vi "GetPlane.vi"(0 "Image In":T1 {"Dialogs" format="%.0b"}) -> (1 "Blue Plane Out":T1 {"Dialogs" format="%.0b"}, 2 "Green Plane Out":T1 {"Dialogs" format="%.0b"}, 3 "Red Plane Out":T1 {"Dialogs" format="%.0b"})   [LabVIEW 2024]
doc: "This VI takes as a 24 bit images as an input and will output three 8 bit channels, one each for Red, Green, and Blue."
uses:
  <userlib>/ImageProcessing/QTLIB_2595_LV86/QT_Image.ctl
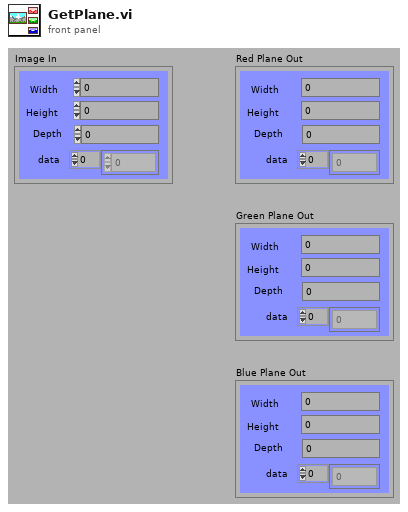
[diagram p1: front panel]
types:
  T1 = typedef "QT_Image.ctl" = cluster{"Width":i32, "Height":i32, "Depth":i32, "data":u8[], "Compressed data":u8[], "Color table":u32[], "Duration":i32, "Options":i32, "Timestamp":i32, "ID":i32, "Reserved":i32, "Dialogs":u32}
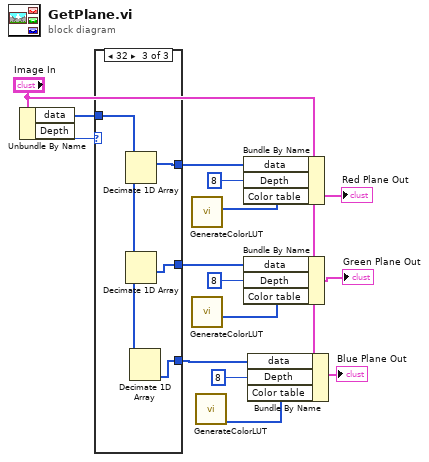
[diagram p0: block diagram]
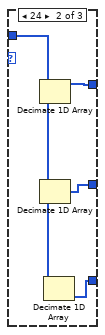
[diagram p3: hidden frame]
diagram:
  n1 = Unbundle By Name("Image In") -> ("data"=w10:u8[], "Depth"=w5:i32)
  n2 = case shown="32" w5 {
    tunnel: [w16 w18 w22] -> w4
    tunnel: w10 -> [w16 w20 w24]
    tunnel: [w16 w19 w23] -> w3
    tunnel: [w16 w17 w21] -> w2
    frame Default {
    }
    frame 24 {
      n3 = Decimate 1D Array(w20) -> (w18:u8[])  [unwired: 2 out]
      n4 = Decimate 1D Array(w20) -> (w19:u8[])  [unwired: 2 out]
      n5 = Decimate 1D Array(w20) -> (w17:u8[])  [unwired: 2 out]
    }
    frame 32 {
      n6 = Decimate 1D Array(w24) -> (w22:u8[])  [unwired: 3 out]
      n7 = Decimate 1D Array(w24) -> (w23:u8[])  [unwired: 3 out]
      n8 = Decimate 1D Array(w24) -> (w21:u8[])  [unwired: 3 out]
    }
  }
  n9 = call <userlib>:"GenerateColorLUT.vi"() -> ("Red"=w13:u32[])  [unwired: 4 out]
  n10 = call <userlib>:"GenerateColorLUT.vi"() -> ("Green"=w9:u32[])  [unwired: 4 out]
  n11 = call <userlib>:"GenerateColorLUT.vi"() -> ("Blue"=w8:u32[])  [unwired: 4 out]
  n12 = Bundle By Name(cluster="Image In", "data"=w4, "Depth"=8, "Color table"=w13) -> (→"Red Plane Out":T1)
  n13 = Bundle By Name(cluster="Image In", "data"=w3, "Depth"=8, "Color table"=w9) -> (→"Green Plane Out":T1)
  n14 = Bundle By Name(cluster="Image In", "data"=w2, "Depth"=8, "Color table"=w8) -> (→"Blue Plane Out":T1)
